vi "writeToXML.vi"(8 "error in (no error)":errorcluster, 10 "Class Label":string, 11 "CableWrapCommands in":refnum<class "CableWrapCommands.lvclass">) -> (0 "error out":errorcluster, 2 "XML out":string, 3 "CableWrapCommands out":refnum<class "CableWrapCommands.lvclass">)   [LabVIEW 2022 SP3, in "TCSDataDefinitions.lvlib" / "TCSCommand.lvlib" / "CableWrapCommands.lvlib" / "CableWrapCommands.lvclass"]
uses:
  CableWrapCommands.lvclass
  CableWrapCommands.lvclass/CableWrapCommands.ctl
  TCSTcsCommand/TCSTcsCommand.lvclass
  <userlib>/Common/XML/XMLGenerator/XMLGenerator.lvclass
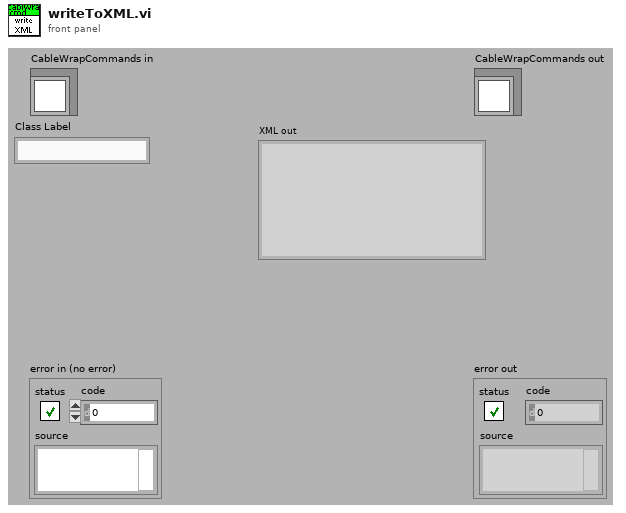
[diagram p1: front panel]
types:
  T1 = typedef "TCSDataDefinitions.lvlib/TCSCommand.lvlib/CableWrapCommands.lvlib/WrapnumTypes.ctl" = enum16{"-1", "0", "1"}
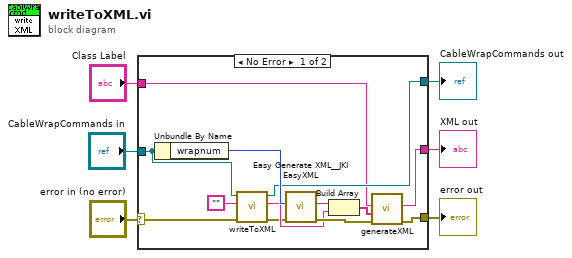
[diagram p0: block diagram]
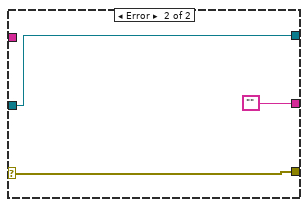
[diagram p2: hidden frame]
diagram:
  n1 = case shown="No Error" "error in (no error)" {
    selector: "error in (no error)" -> [w8 w20]
    tunnel: [w12 w22] -> w4
    tunnel: "CableWrapCommands in" -> [w13 w22]
    tunnel: [w14 ""] -> w3
    tunnel: [w15 w20] -> w2
    tunnel: "Class Label" -> [w10 _]
    frame No Error {
      n2 = Unbundle By Name(w13) -> ("wrapnum"=w19:T1)
      n3 = call-parent "writeToXML.vi"("error in (no error)"=w8, "ClassLabel"="", "TCSTcsCommand in"=w13) -> ("error out"=w7:errorcluster, "XML out"=w11:string, "TCSTcsCommand out"=w12:refnum<class "CableWrapCommands.lvclass">)  [unwired: 6 in]
      n4 = call <vilib>:"Easy Generate XML__JKI EasyXML.vi"("error in (no error)"=w7, "LabVIEW Data"=w19) -> ("error out"=w16:errorcluster, "XML String"=w18:string)  [unwired: 8 in]
      n5 = Build Array(w18, w11) -> (w17:string[])
      n6 = call <userlib>:"generateXML.vi"("error in"=w16, "childrenXML"=w17, "elementName"=w10) -> ("error out"=w15:errorcluster, "XML out"=w14:string)  [unwired: 6 in, 1 out]
    }
    frame Error {
    }
  }
  "error out" <- w2
  "CableWrapCommands out" <- w4
  "XML out" <- w3
